vi "PrepareForRun.vi"(8 "ErrorIn":errorcluster, 11 "YActorIn":refnum<class "YActor.lvclass">) -> (0 "ErrorOut":errorcluster, 3 "YActorOut":refnum<class "YActor.lvclass">)   [LabVIEW 2021, in "YActor.lvclass"]
uses:
  YActor.lvclass
  YActor.lvclass/YActor.ctl
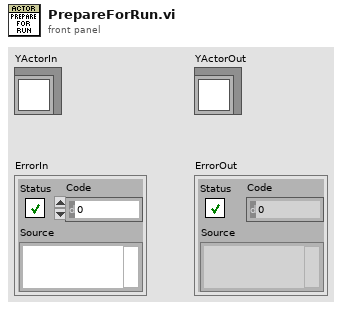
[diagram p1: front panel]
types:
  T1 = cluster{"UIEvent":cluster{"Event":string, "This":refnum<class>, "Data":variant}}
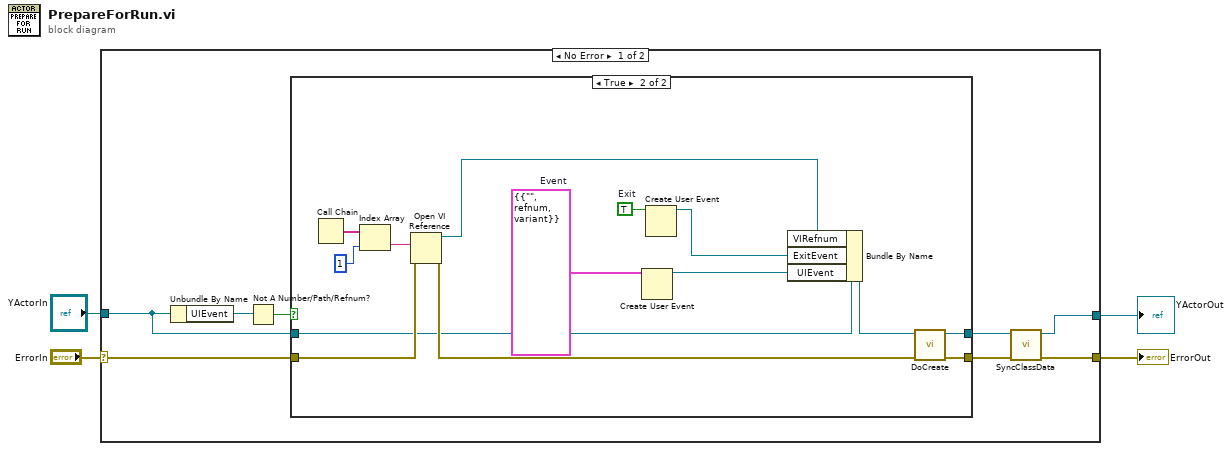
[diagram p0: block diagram]
diagram:
  n1 = case shown="No Error" "ErrorIn" {
    selector: "ErrorIn" -> [w12 w30]
    tunnel: "YActorIn" -> [w9 w29]
    tunnel: [w5 w29] -> w1
    tunnel: [w10 w30] -> w4
    frame No Error {
      n2 = Unbundle By Name(w9) -> ("UIEvent"=w8:refnum<user-event>)
      n3 = Not A Number/Path/Refnum?(number/path/refnum=w8) -> (NaN/Path/Refnum?=w7:bool)
      n4 = case shown="True" w7 {
        tunnel: [w13 w24] -> w6
        tunnel: w9 -> [w13 w23]
        tunnel: w12 -> [w14 w26]
        tunnel: [w14 w28] -> w11
        frame False {
          # "This part is called when the class is derived"
        }
        frame True {
          w19 = T1 {"UIEvent"={"Event"="", "This"=refnum, "Data"=variant}}  # Event
          w25 = TRUE  # Exit
          n5 = Call Chain() -> (call chain=w18:string[])
          n6 = Index Array(array=w18, index=1) -> (element=w16:string)
          n7 = Open VI Reference(vi path=w16, error in (no error)=w26) -> (vi reference=w15:refnum<vi>, error out=w27:errorcluster)  [unwired: 4 in]
          n8 = Create User Event(user event datatype=w19) -> (user event=w20:refnum<user-event>)  [unwired: 1 in, 1 out]
          n9 = Create User Event(user event datatype=w25) -> (user event=w21:refnum<user-event>)  [unwired: 1 in, 1 out]
          n10 = Bundle By Name(cluster=w23, "VIRefnum"=w15, "ExitEvent"=w21, "UIEvent"=w20) -> (w22:refnum<class "YActor.lvclass">)
          n11 = call-dynamic "DoCreate.vi"("ErrorIn"=w27, "YActor in"=w22) -> ("ErrorOut"=w28:errorcluster, "YActor out"=w24:refnum<class "YActor.lvclass">)  [unwired: 8 in]
        }
      }
      n12 = call "SyncClassData.vi"("error in (no error)"=w11, "YActor in"=w6) -> ("error out"=w10:errorcluster, "YActor out"=w5:refnum<class "YActor.lvclass">)  [unwired: 8 in]
    }
    frame Error {
    }
  }
  "YActorOut" <- w1
  "ErrorOut" <- w4
